vi "transmitRFID.vi"() -> ()   [LabVIEW 2015]
uses:
  Global_bits.vi
  <instrlib>/niUSRP/niUSRP Write Tx Data (CDB).vi
panel:
  out "RN16 array":i32[](array[numeric])
  out "size(s)":i32
  out "Bits Graph":i16[](graph)
  out "error out":errorcluster
  in  "RFID":bool
  in  "Parameters Query":T1 {"Session" items=["S0", "S1", "S2", "S3"]; "Sel" items=["All", "All2", "~SL", "SL"]; "M" items=["M=1", "M=2", "M=4", "M=8"]}
  out "Waveform Magnitude":dbl[](graph)
  out "Samples":i32
  out "Loop":i32
  in  "Symbol Rate [Hz]":dbl=500000.0 format="%#_13p"
  in  "Parameters Select":T2={"Target"=7, "Action"=0, "MemBank"=1, "truncate"=FALSE} {"MemBank" items=["00 RFU", "01 EPC", "10 TID", "11 User"]; "Action" items=["000", "001", "010", "011", "100", "101", "110", "111"]; "Target" items=["000 Inventoried (S0)", "001 Inventoried (S1)", "010 Inventoried (S2)", "011 Inventoried (S3)", "100 SL", "101 RFU", "110 RFU", "111 RFU"]}
  in  "Parameters Symbols":T3={"Tari"=8e-06, "PW"=0.5, "factor for \"1\" symbol"=0.5, "RTcal"=2.5, "TRcal"=3.0, "Delimiter"=1.25e-05} {"TRcal" min=1.1 max=3.0 step=0.1; "RTcal" min=2.5 max=3.0 step=0.1; "factor for \"1\" symbol" min=0.5 max=1.0 step=0.1; "PW" min=0.265 max=0.525 step=0.001; "Tari" format="%#_3p"}
  out "coerced IQ rate":dbl=100000.0 format="%#_6p"
  out "carrier frequency":dbl=100000.0 format="%#_6p"
  out "coerced gain":dbl format="%#_6f"
  in  "stop":bool
  in  "IQ rate":dbl=2000000.0 format="%#_6p"
  in  "carrier frequency":dbl=920000000.0 format="%#_6p"
  in  "gain":dbl format="%#_6f"
  in  "tx device names":refnum<k15>="192.168.20.13"
  # "Transmit RFID"
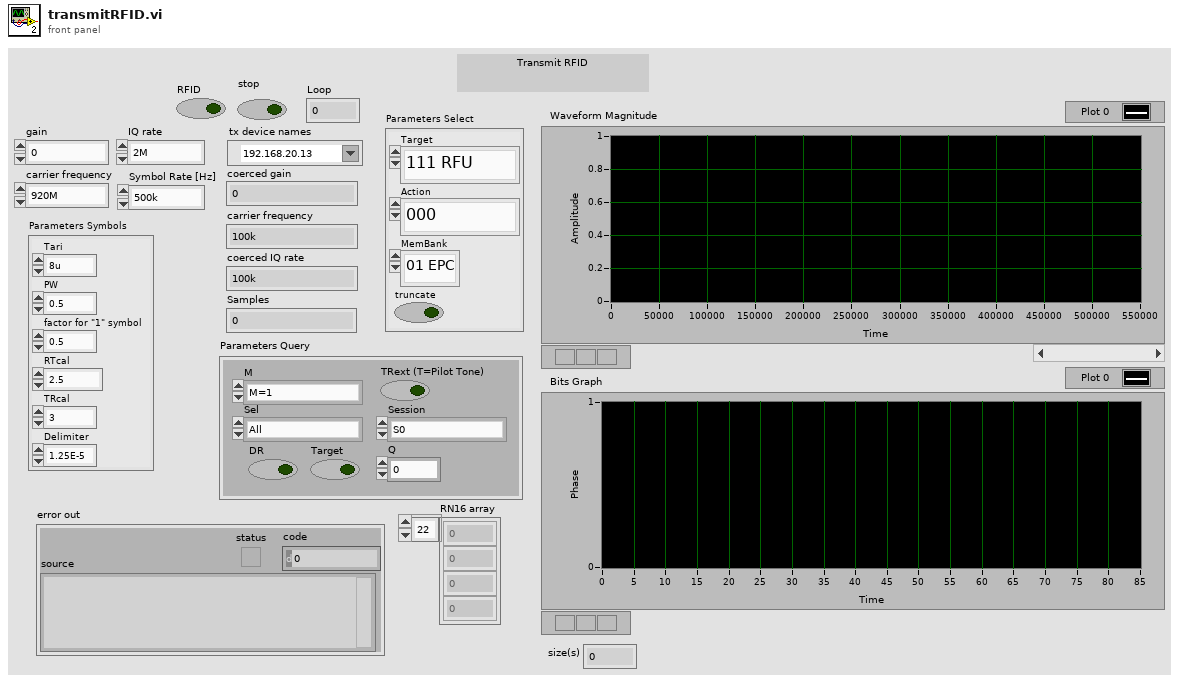
[diagram p1: front panel]
types:
  T1 = cluster{"DR":bool, "M":u16, "TRext (T=Pilot Tone)":bool, "Sel":u16, "Session":u16, "Q":u8, "Target":bool}
  T2 = cluster{"Target":u16, "Action":u16, "MemBank":u16, "truncate":bool}
  T3 = cluster{"Tari":dbl, "PW":dbl, "factor for \"1\" symbol":dbl, "RTcal":dbl, "TRcal":dbl, "Delimiter":dbl}
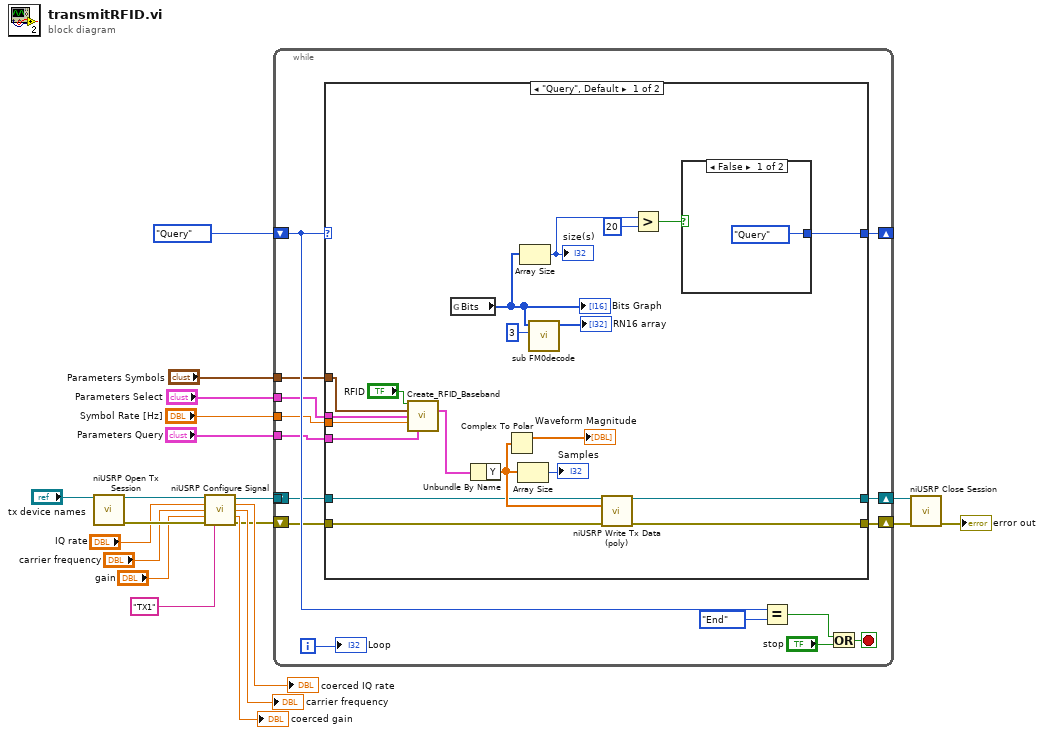
[diagram p0: block diagram]
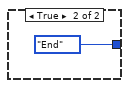
[diagram p2: hidden frame]
diagram:
  n1 = call <instrlib>:"niUSRP Open Tx Session.vi"("device names"="tx device names") -> ("session handle out"=w8:refnum<k15>, "error out"=w20:errorcluster)  [unwired: 13 in]
  n2 = call <instrlib>:"niUSRP Configure Signal.vi"("session handle"=w8, "IQ rate"="IQ rate", "carrier frequency"="carrier frequency", "gain"="gain", "error in (no error)"=w20, "active antenna"="TX1") -> ("session handle out"=w6:refnum<k15>, "coerced IQ rate"=→"coerced IQ rate":dbl, "coerced carrier frequency"=→"carrier frequency":dbl, "coerced gain"=→"coerced gain":dbl, "error out"=w5:errorcluster)  [unwired: 5 in]
  n3 = while {
    tunnel: "Parameters Symbols" -> [w25]
    tunnel: "Parameters Select" -> [w24]
    tunnel: "Symbol Rate [Hz]" -> [w23]
    tunnel: "Parameters Query" -> [w22]
    tunnel: w6 -> [w29]
    shift-right: [w27] -> w4
    shift-left: w5 -> [w28]
    shift-right: [w26] -> w1
    shift-left: _ -> [_]
    shift-right: [w21] -> _
    shift-left: enum16{"Query", "End"}."Query" -> [w30]
    i -> [w34]
    stop <- w33 stop-if-true
    n4 = case shown="\"Query\", Default" w30 {
      selector: w30 -> [_ w58]
      tunnel: w29 -> [w50 w60]
      tunnel: w28 -> [w49 w59]
      tunnel: [w48 w59] -> w27
      tunnel: [w47 w60] -> w26
      tunnel: w25 -> [w46 _]
      tunnel: w24 -> [w45 _]
      tunnel: w23 -> [w44 _]
      tunnel: w22 -> [w43 _]
      tunnel: [w37 w58] -> w21
      frame "Query", Default {
        n5 = call "Create_RFID_Baseband.vi"("RFID"="RFID", "Parameters Symbols"=w46, "Parameters Select"=w45, "Symbol Rate [Hz]"=w44, "Parameters Query"=w43) -> ("complex waveform"=w53:cluster{"t0":dbl, "dt":dbl, "Y":cdb[]})  [unwired: 9 in, 1 out]
        n6 = global read "Global_bits.vi" "Bits"() -> (w41:i16[])
        "Bits Graph" <- w41
        n7 = Unbundle By Name(w53) -> ("Y"=w51:cdb[])
        n8 = Complex To Polar(r * e^(i*theta)=w51) -> (r=→"Waveform Magnitude":dbl[])  [unwired: 1 out]
        n9 = Array Size(array=w51) -> (size(s)=→"Samples":i32)
        n10 = Array Size(array=w41) -> (size(s)=w40:i32)
        "size(s)" <- w40
        n11 = call "sub FM0decode.vi"("threshold"=3, "Bit Sequence"=w41) -> ("RN16 array"=→"RN16 array":i32[])  [unwired: 9 in]
        n12 = call-poly <instrlib>:"niUSRP Write Tx Data (poly).vi"("session handle"=w50, "data"=w51, "error in (no error)"=w49) -> ("session handle out"=w47:refnum<k15>, "error out"=w48:errorcluster)  [unwired: 11 in]
        n13 = Greater?(x=w40, y=20) -> (0:w38:bool)
        n14 = case shown="False" w38 {
          tunnel: [enum16{"Query", "End"}."Query" enum16{"Query", "End"}."End"] -> w37
          frame False {
          }
          frame True {
          }
        }
      }
      frame "End" {
      }
    }
    n15 = Equal?(x=w30, y=enum16{"Query", "End"}."End") -> (x = y?=w32:bool)
    n16 = Or(x=w32, y="stop") -> (x .or. y?=w33:bool)
    "Loop" <- w34
  }
  n17 = call <instrlib>:"niUSRP Close Session.vi"("session handle"=w1, "error in (no error)"=w4) -> ("error out"=→"error out":errorcluster)  [unwired: 13 in]
